vi "电流解析.vi"(8 "error in":errorcluster caption="错误输入", 11 "Channel":u16=81 format="%.0x") -> (0 "error out":errorcluster caption="错误输出", 3 "读取电流":dbl)   [LabVIEW 2020]
uses:
  D/Program Files (x86)/National Instruments/LabVIEW 2020/user.lib/PCANBasic/PCANBasic.lvlib
panel:
  out "function return 2":u32 format="%.0x"
  out "function return 3":u32 format="%.0x"
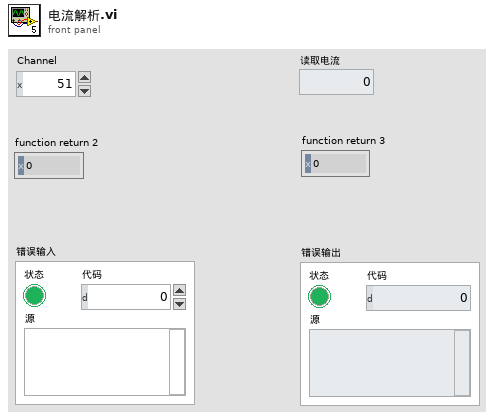
[diagram p1: front panel]
types:
  T1 = cluster{"ID":u32, "MSGTYPE":u8, "DLC":u8, "DATA[0]":u8, "DATA[1]":u8, "DATA[2]":u8, "DATA[3]":u8, "DATA[4]":u8, "DATA[5]":u8, "DATA[6]":u8, "DATA[7]":u8, "DATA[8]":u8, "DATA[9]":u8, "DATA[10]":u8, "DATA[11]":u8, "DATA[12]":u8, "DATA[13]":u8, "DATA[14]":u8, "DATA[15]":u8, "DATA[16]":u8, "DATA[17]":u8, "DATA[18]":u8, "DATA[19]":u8, "DATA[20]":u8, "DATA[21]":u8, "DATA[22]":u8, "DATA[23]":u8, "DATA[24]":u8, "DATA[25]":u8, "DATA[26]":u8, "DATA[27]":u8, "DATA[28]":u8, "DATA[29]":u8, "DATA[30]":u8, "DATA[31]":u8, "DATA[32]":u8, "DATA[33]":u8, "DATA[34]":u8, "DATA[35]":u8, "DATA[36]":u8, "DATA[37]":u8, "DATA[38]":u8, "DATA[39]":u8, "DATA[40]":u8, "DATA[41]":u8, "DATA[42]":u8, "DATA[43]":u8, "DATA[44]":u8, "DATA[45]":u8, "DATA[46]":u8, "DATA[47]":u8, "DATA[48]":u8, "DATA[49]":u8, "DATA[50]":u8, "DATA[51]":u8, "DATA[52]":u8, "DATA[53]":u8, "DATA[54]":u8, "DATA[55]":u8, "DATA[56]":u8, "DATA[57]":u8, "DATA[58]":u8, "DATA[59]":u8, "DATA[60]":u8, "DATA[61]":u8, "DATA[62]":u8, "DATA[63]":u8}
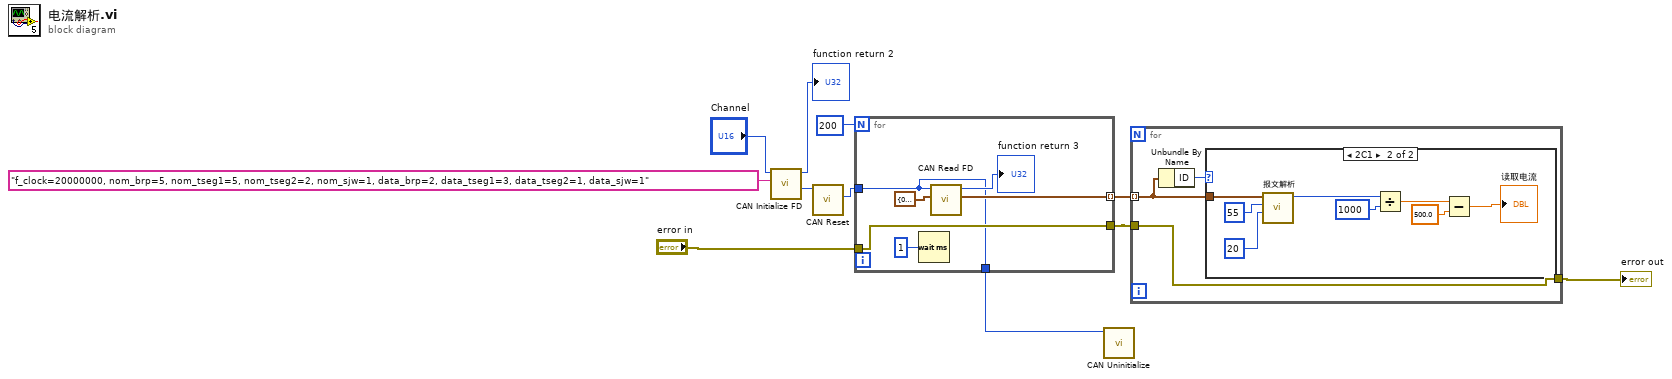
[diagram p0: block diagram]
diagram:
  n1 = call "CAN Initialize FD.vi"("BitrateFD"="f_clock=20000000, nom_brp=5, nom_tseg1=5, nom_tseg2=2, nom_sjw=1, data_brp=2, data_tseg1=3, data_tseg2=1, data_sjw=1", "Channel"="Channel") -> ("Channel out"=w7:u16, "function return"=→"function return 2":u32)  [unwired: 7 in, 1 out]
  n2 = call "CAN Reset.vi"("Channel in"=w7) -> ("Channel out"=w2:u16)  [unwired: 9 in, 1 out]
  n3 = for {
    N: 200 -> [_]
    tunnel: w2 -> [w12]
    tunnel: [w14] -> w6 mode=indexing
    tunnel: "error in" -> [w13]
    tunnel: [w13] -> w4
    tunnel: [w12] -> w1
    n4 = Wait (ms)(milliseconds to wait=u32 1 ("等待时间（毫秒）")) -> ()  [unwired: 1 out]
    n5 = call "CAN Read FD.vi"("MessageBuffer"=T1 {"ID"=0, "MSGTYPE"=0, "DLC"=0, "DATA[0]"=0, "DATA[1]"=0, "DATA[2]"=0, "DATA[3]"=0, "DATA[4]"=0, "DATA[5]"=0, "DATA[6]"=0, "DATA[7]"=0, "DATA[8]"=0, "DATA[9]"=0, "DATA[10]"=0, "DATA[11]"=0, "DATA[12]"=0, "DATA[13]"=0, "DATA[14]"=0, "DATA[15]"=0, "DATA[16]"=0, "DATA[17]"=0, "DATA[18]"=0, "DATA[19]"=0, "DATA[20]"=0, "DATA[21]"=0, "DATA[22]"=0, "DATA[23]"=0, "DATA[24]"=0, "DATA[25]"=0, "DATA[26]"=0, "DATA[27]"=0, "DATA[28]"=0, "DATA[29]"=0, "DATA[30]"=0, "DATA[31]"=0, "DATA[32]"=0, "DATA[33]"=0, "DATA[34]"=0, "DATA[35]"=0, "DATA[36]"=0, "DATA[37]"=0, "DATA[38]"=0, "DATA[39]"=0, "DATA[40]"=0, "DATA[41]"=0, "DATA[42]"=0, "DATA[43]"=0, "DATA[44]"=0, "DATA[45]"=0, "DATA[46]"=0, "DATA[47]"=0, "DATA[48]"=0, "DATA[49]"=0, "DATA[50]"=0, "DATA[51]"=0, "DATA[52]"=0, "DATA[53]"=0, "DATA[54]"=0, "DATA[55]"=0, "DATA[56]"=0, "DATA[57]"=0, "DATA[58]"=0, "DATA[59]"=0, "DATA[60]"=0, "DATA[61]"=0, "DATA[62]"=0, "DATA[63]"=0}, "Channel"=w12) -> ("MessageBuffer out"=w14:T1, "function return"=→"function return 3":u32)  [unwired: 6 in, 2 out]
  }
  n6 = call "CAN Uninitialize.vi"("Channel"=w1) -> ()  [unwired: 10 in, 1 out]
  n7 = for {
    tunnel: w6 -> [w19] mode=indexing
    tunnel: w4 -> [w18]
    tunnel: [w18] -> w3
    n8 = Unbundle By Name(w19) -> ("ID"=w20:u32)
    n9 = case shown="2C1" w20 {
      tunnel: w19 -> [_ w28]
      frame 0, Default {
      }
      frame 705 {
        n10 = call "报文解析.vi"("长度"=20, "起始位"=55, "MessageBuffer"=w28) -> ("数字"=w25:u32)  [unwired: 8 in]
        n11 = Divide(x=w25, y=u32 1000) -> (x/y=w23:dbl)
        n12 = Subtract(x=w23, y=500.0) -> (x-y=→"读取电流":dbl)
      }
    }
  }
  "error out" <- w3
